vi "Get Server Configuration.vi"(8 "error in (no error)":errorcluster) -> (0 "error out":errorcluster, 2 "Subsystem I/O Attributes":T1[](array[typedef]), 3 "System Configuration":T4)   [LabVIEW 2024]
doc: "Gets current server configurations."
uses:
  Controls/Server/System Configuration.ctl
  Controls/Server/Subsystem Configuration.ctl
  Controls/Server/Subsystem IO Attributes.ctl
  Controls/Server/Subsystem IO Logging Attributes.ctl
  Controls/Server/Subsystem IO Alarm Attributes.ctl
  Globals/Global - Server.vi
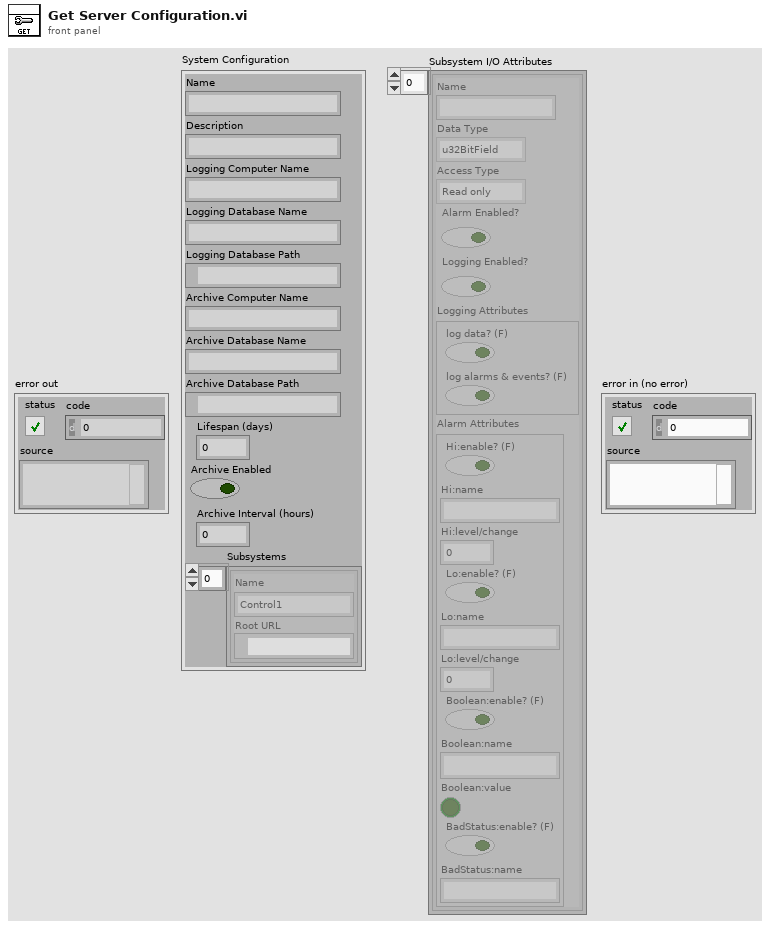
[diagram p1: front panel]
types:
  T1 = typedef "Subsystem IO Attributes.ctl" = cluster{"Name":string, "Data Type":enum32{"u32BitField", "bool", "double", "string", "int8", "uint8", "int16", "uint16", "int32", "uint32", "int64", "uint64", "single", "double waveform", "int16 waveform", "array of boolean", "array of int8", "array of uint8", "array of int16", "array of uint16", "array of int32", "array of uint32", "array of int64", "array of uint64", "array of single", "array of double", "array of double waveform", "array of int16 waveform", "array of string", "variant", "timestamp", "fixed point", "custom"}, "Access Type":enum32{"Read only", "Write only", "Read/write"}, "Alarm Enabled?":bool, "Logging Enabled?":bool, "Logging Attributes":T2, "Alarm Attributes":T3}
  T2 = typedef "Subsystem IO Logging Attributes.ctl" = cluster{"log data? (F)":bool, "log alarms & events? (F)":bool}
  T3 = typedef "Subsystem IO Alarm Attributes.ctl" = cluster{"Hi:enable? (F)":bool, "Hi:name":string, "Hi:level/change":dbl, "Lo:enable? (F)":bool, "Lo:name":string, "Lo:level/change":dbl, "Boolean:enable? (F)":bool, "Boolean:name":string, "Boolean:value":bool, "BadStatus:enable? (F)":bool, "BadStatus:name":string}
  T4 = typedef "System Configuration.ctl" = cluster{"Name":string, "Description":string, "Logging Computer Name":string, "Logging Database Name":string, "Logging Database Path":path, "Archive Computer Name":string, "Archive Database Name":string, "Archive Database Path":path, "Lifespan (days)":u32, "Archive Enabled":bool, "Archive Interval (hours)":u32, "Subsystems":T5[]}
  T5 = typedef "Subsystem Configuration.ctl" = cluster{"Name":string, "Root URL":refnum<k21>}
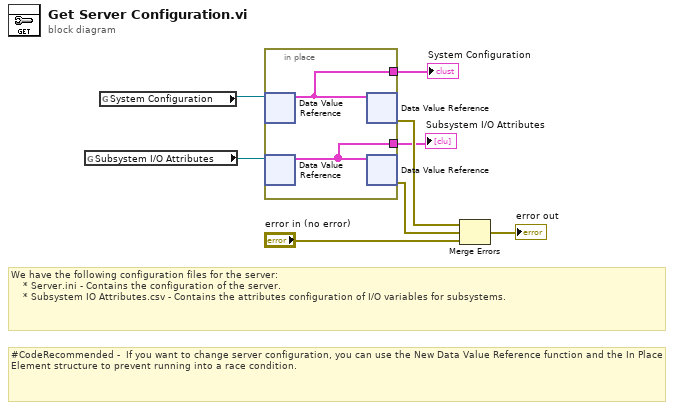
[diagram p0: block diagram]
diagram:
  # "#CodeRecommended -  If you want to change server configuration, you can use the New Data Value Reference function and the In Place Element structure to prevent running into a race condition."
  # "We have the following configuration files for the server:\n    * Server.ini - Contains the configuration of the server.\n    * Subsystem IO Attributes.csv - Contains the attributes configuration of I/O variables for subsystems."
  n1 = global read "Global - Server.vi" "Subsystem I/O Attributes"() -> (w3:refnum<data-value>)
  n2 = global read "Global - Server.vi" "System Configuration"() -> (w8:refnum<data-value>)
  n3 = in-place {
    in-place-border: [w10] -> w7
    in-place-border: [w9] -> w1
    n4 = in-place-dvr #1(w8) -> (w10:T4)  [unwired: 1 out]
    n5 = in-place-dvr #2(w3) -> (w9:T1[])  [unwired: 1 out]
    n6 = in-place-dvr #1(w10) -> (w6:errorcluster)  [unwired: 1 out]
    n7 = in-place-dvr #2(w9) -> (w2:errorcluster)  [unwired: 1 out]
  }
  "System Configuration" <- w7
  "Subsystem I/O Attributes" <- w1
  n8 = Merge Errors(w6, w2, "error in (no error)") -> (→"error out":errorcluster)
